vi "Receiving Modulated Audio.vi"() -> ()   [LabVIEW 2019]
doc: "This application receives an audio modulated signal from the other target by communicating with a TCP protocol. The signal is then outputed through the EMONA Communications Board for its demodulation. After being demodulated, the signal is reproduced on the headphones and inputed once again to the application. Finally the application displays the message received through the Message Chart."
uses:
  <vilib>/myRIO/Instrument Drivers/Onboard IO/AO Continuous/typedefs/AO Continuous Reference.ctl
  <vilib>/myRIO/Common/Instrument Driver Framework/Utilities/typedefs/myRIO Generic Hardware Reference.ctl
  <vilib>/myRIO/Common/Instrument Driver Framework/Utilities/typedefs/Hardware Version Enum.ctl
  <vilib>/myRIO/Common/Instrument Driver Framework/Utilities/typedefs/myRIO v1.0 Reference.ctl
  <vilib>/myRIO/Common/Instrument Driver Framework/Utilities/typedefs/Generic FPGA Reference.ctl
  <vilib>/myRIO/Common/Instrument Driver Framework/ELVIS III v1.0/AO Continuous/typedefs/AO Continuous Channels List.ctl
  <vilib>/myRIO/Common/Instrument Driver Framework/ELVIS III v1.0/AO Continuous/typedefs/ELVIS III v1.0 AO Continuous Channels Enum.ctl
  <vilib>/myRIO/Common/Instrument Driver Framework/ELVIS III v1.0/AO Continuous/typedefs/AO Continuous Channel Info.ctl
  <vilib>/userDefined/High Color/nirio_resource_hc.ctl
  <vilib>/myRIO/Instrument Drivers/Onboard IO/AI Block/typedefs/AI Block Reference.ctl
  <vilib>/myRIO/Common/Instrument Driver Framework/myRIO v1.0/AI Block/typedefs/AI Block Channels List.ctl
  <vilib>/myRIO/Common/Instrument Driver Framework/myRIO v1.0/AI Block/typedefs/AI Block Channels Enum.ctl
  <vilib>/myRIO/Common/Instrument Driver Framework/Utilities/typedefs/Analog Scaling Constants.ctl
  <vilib>/myRIO/Common/Instrument Driver Framework/ELVIS III v1.0/AO Continuous/vis/ELVIS III v1.1 Open AO (Continuous).vi
  <vilib>/myRIO/Common/Instrument Driver Framework/ELVIS III v1.0/AI Block/vis/ELVIS III v1.1 Open AI (N Samples).vi
  <vilib>/myRIO/Common/Instrument Driver Framework/Utilities/vis/Validate Channels.vi
  <vilib>/myRIO/Common/Instrument Driver Framework/ELVIS III v1.0/AO Continuous/vis/ELVIS III v1.0 Reserve AO Continuous.vi
  <vilib>/myRIO/Common/Instrument Driver Framework/ELVIS III v1.0/Resource Manager/vis/ELVIS III v1.0 Check For Different Banks.vi
  <vilib>/myRIO/Common/Instrument Driver Framework/ELVIS III v1.0/AI Block/vis/ELVIS III v1.0 AI Block Read.vi
  <vilib>/myRIO/Common/Instrument Driver Framework/ELVIS III v1.0/AI Block/vis/ELVIS III v1.0 Close AI Block.vi
  <vilib>/myRIO/Common/Instrument Driver Framework/ELVIS III v1.0/AO Continuous/vis/ELVIS III v1.1 Close AO Continuous.vi
  <vilib>/myRIO/Common/Instrument Driver Framework/myRIO v1.0/UART/vis/myRIO v1.0 Close UART.vi
  <vilib>/myRIO/Common/Instrument Driver Framework/ELVIS III v1.0/AO Continuous/vis/ELVIS III v1.0 Build MUX Configuration AO Continuous.vi
  <vilib>/myRIO/Common/Instrument Driver Framework/Utilities/vis/Sample Rate To Ticks.vi
  <vilib>/myRIO/Common/Instrument Driver Framework/ELVIS III v1.0/AI Block/vis/ELVIS III v1.0 Unreserve AI Block.vi
  <vilib>/myRIO/Common/Instrument Driver Framework/ELVIS III v1.0/AO Continuous/vis/ELVIS III v1.0 Unreserve AO Continuous.vi
  <vilib>/myRIO/Common/Instrument Driver Framework/ELVIS III v1.0/AI Block/vis/ELVIS III v1.0 Build MUX Configuration AI Block.vi
  <vilib>/Utility/VariantDataType/GetNumericInfo.vi
  <vilib>/Utility/error.llb/Error Cluster From Error Code.vi
  <vilib>/myRIO/Common/Instrument Driver Framework/ELVIS III v1.0/ELVIS III v1.1 Open.vi
  <vilib>/myRIO/Common/Instrument Driver Framework/ELVIS III v1.0/Resource Manager/vis/ELVIS III v1.0 Coerce AI Scaling.vi
  <vilib>/myRIO/Common/Instrument Driver Framework/ELVIS III v1.0/AI Block/vis/ELVIS III v1.0 Reserve AI Block.vi
  <vilib>/myRIO/Common/Instrument Driver Framework/ELVIS III v1.0/Resource Manager/vis/ELVIS III v1.0 Configure DMAs.vi
  <vilib>/myRIO/Common/Instrument Driver Framework/myRIO v1.0/myRIO v1.0 Close.vi
  <vilib>/myRIO/Common/Instrument Driver Framework/ELVIS III v1.0/Resource Manager/vis/ELVIS III v1.0 Reserve Channel List.vi
  <vilib>/myRIO/Common/Instrument Driver Framework/ELVIS III v1.0/AO Continuous/vis/ELVIS III v1.1 Stop AO Continuous.vi
  <vilib>/myRIO/Common/Instrument Driver Framework/myRIO v1.0/Resource Manager/vis/myRIO v1.0 Block Write Configuration.vi
  <vilib>/myRIO/Common/Instrument Driver Framework/ELVIS III v1.0/AI Block/vis/ELVIS III v1.0 AI Block Read Bank A.vi
  <vilib>/myRIO/Common/Instrument Driver Framework/ELVIS III v1.0/AI Block/vis/ELVIS III v1.0 AI Block Read Bank B.vi
  <vilib>/myRIO/Common/Instrument Driver Framework/ELVIS III v1.0/AO Continuous/vis/ELVIS III v1.0 AO Continuous Write.vi
  <vilib>/myRIO/Common/Instrument Driver Framework/ELVIS III v1.0/AO Continuous/vis/ELVIS III v1.1 Start AO Continuous.vi
  <vilib>/myRIO/Common/Instrument Driver Framework/ELVIS III v1.0/Resource Manager/vis/ELVIS III v1.0 Unreserve Channel List.vi
  <vilib>/myRIO/Common/Instrument Driver Framework/Utilities/vis/FPGA Ref Manager.vi
  <vilib>/myRIO/Common/Instrument Driver Framework/ELVIS III v1.0/ELVIS III v1.0 Reset FPGA.vi
  <vilib>/myRIO/Common/Instrument Driver Framework/myRIO v1.0/IRQ/vis/myRIO v1.0 IRQ Info FGV.vi
  <vilib>/myRIO/Common/Instrument Driver Framework/myRIO v1.0/IRQ/vis/myRIO v1.0 Timer IRQ Info FGV.vi
  <vilib>/myRIO/Common/Instrument Driver Framework/myRIO v1.0/IRQ/vis/myRIO v1.0 ISR Agent.vi
  <vilib>/myRIO/Instrument Drivers/Utilities/vis/Reset Index.vi
  <vilib>/myRIO/Common/Instrument Driver Framework/myRIO v1.0/Resource Manager/vis/myRIO v1.0 Block Write Resource Manager.vi
  <vilib>/myRIO/Instrument Drivers/Onboard IO/AI Block/vis/myRIO AI N Samples Open.xnode
  <vilib>/myRIO/Instrument Drivers/Onboard IO/AO Continuous/vis/myRIO AO Continuous Open.xnode
  <vilib>/myRIO/Instrument Drivers/Utilities/Utilities.lvlib
  <vilib>/myRIO/Instrument Drivers/Onboard IO/AI Block/AI Block.lvlib
  <vilib>/myRIO/Instrument Drivers/Onboard IO/AO Continuous/AO Continuous.lvlib
panel:
  out "Demodulator":string caption="Demodulator IP Address"
  out "Message":dbl[](graph)
  out "Signal":dbl[](graph) caption="Modulated Signal"
  out "Error Out":errorcluster
  in  "Stop":bool
  # "Receiving and Demodulating Audio"
  # "Explanation:\nThis application receives an audio modulated signal from the other target by communicating with a TCP protocol. The signal is then outputed through the EMONA Communications Board for its demodulation. After being demodulated, the signal is reproduced on the headphones and inputed once again to the application. Finally the application displays the message received through the Message Chart.\n \nThe audio from the target might sound lightly distortioned because of the modulation and demodulation process that was applied to the signal.\n \nInstructions:\n •  Make sure that you have uploaded at least one audio file to the Modulating target for its reproduction (use the Uploading Audio Files VI to do this).\n • Deploy the matching VIs (Sending and Receiving) to each target.\n • Enter the text from the indicator below into the Demodulator IP Address control from the Sending Modulated Audio.vi.\n • Run this VI again and afterwards run the other VI.\n • Try changing between songs and hearing the audio from both targets.\n • If you are not going to use any of the VIs from this project anymore, run the Remove Audio Files VI on the other target."
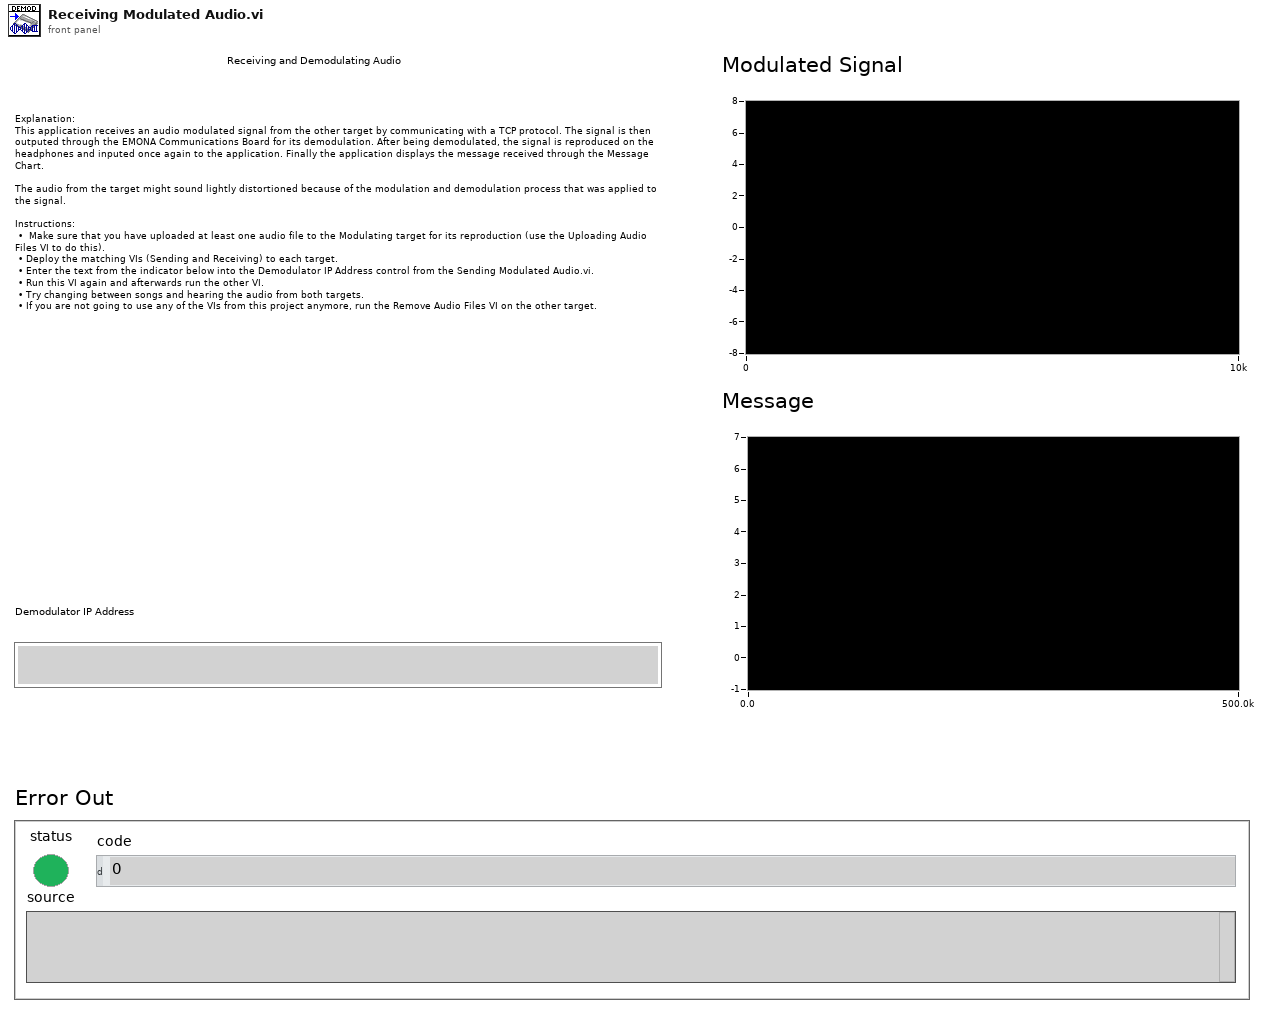
[diagram p1: front panel]
types:
  T1 = typedef "AO Continuous.lvlib/AO Continuous Reference.ctl" = cluster{"myRIO Reference":T2, "AO (Continuous) Channels List":T6, "Channel Info":T8}
  T2 = typedef "myRIO Generic Hardware Reference.ctl" = cluster{"myRIO Model":T3, "myRIO Hardware Reference":T4}
  T3 = typedef "Hardware Version Enum.ctl" = enum16{"Unknown", "myRIO-1900", "myRIO-1950", "roboRIO", "NI ELVIS RIO CM", "ELVIS III"}
  T4 = typedef "myRIO v1.0 Reference.ctl" = cluster{"Generic FPGA Reference":T5, "Allow multiple opens":bool}
  T5 = typedef "Generic FPGA Reference.ctl" = refnum<k20>
  T6 = typedef "AO Continuous Channels List.ctl" = T7[]
  T7 = typedef "ELVIS III v1.0 AO Continuous Channels Enum.ctl" = enum16{"Not Connected", "A/AO0 (Continuous)", "A/AO1 (Continuous)", "B/AO0 (Continuous)", "B/AO1 (Continuous)"}
  T8 = typedef "AO Continuous Channel Info.ctl" = cluster{"Channel Bitmask":u8[], "Channel Index":i32[], "Channel Number":u8}
  T9 = typedef "AI Block.lvlib/AI Block Reference.ctl" = cluster{"myRIO Reference":T2, "AI (N Samples) Channels List":T10, "AI (N Samples) Scaling Constants List":T12[]}
  T10 = typedef "AI Block Channels List.ctl" = T11[]
  T11 = typedef "AI Block Channels Enum.ctl" = enum16{"Not Connected", "A/AI0 (N Samples)", "A/AI1 (N Samples)", "A/AI2 (N Samples)", "A/AI3 (N Samples)", "A/AI4 (N Samples)", "A/AI5 (N Samples)", "A/AI6 (N Samples)", "A/AI7 (N Samples)", "A/AI0 (DIFF N Samples)", "A/AI1 (DIFF N Samples)", "A/AI2 (DIFF N Samples)", "A/AI3 (DIFF N Samples)", "B/AI0 (N Samples)", "B/AI1 (N Samples)", "B/AI2 (N Samples)", "B/AI3 (N Samples)", "B/AI4 (N Samples)", "B/AI5 (N Samples)", "B/AI6 (N Samples)", "B/AI7 (N Samples)", "B/AI0 (DIFF N Samples)", "B/AI1 (DIFF N Samples)", "B/AI2 (DIFF N Samples)", "B/AI3 (DIFF N Samples)"}
  T12 = typedef "Analog Scaling Constants.ctl" = cluster{"LSB Weight (Volts)":dbl, "Offset (Volts)":dbl, "Signed?":bool}
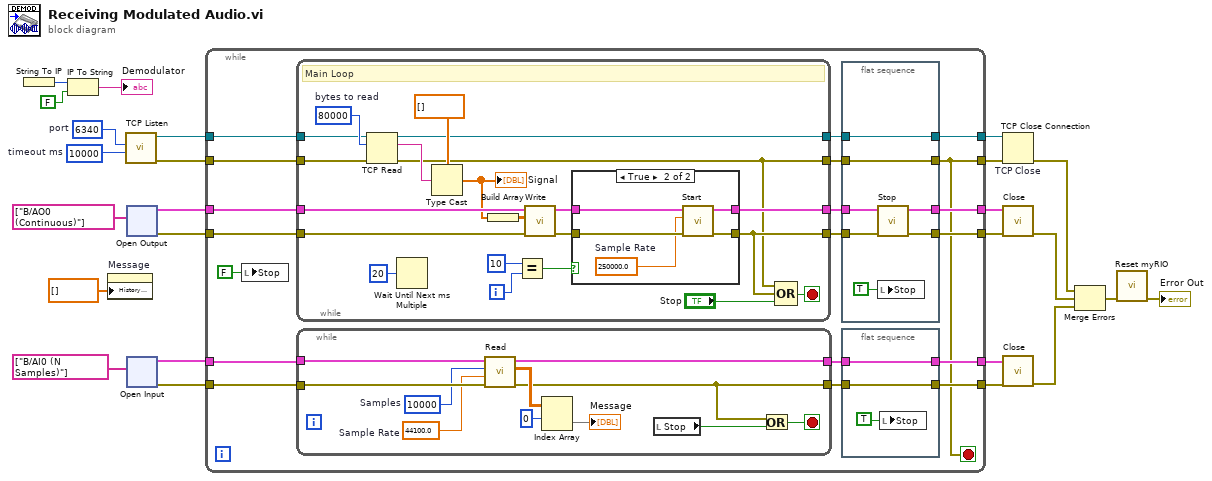
[diagram p0: block diagram]
diagram:
  w7 = 10000  # timeout ms
  w8 = u16 6340  # port
  n1 = String To IP() -> (0:w10:u32)  [unwired: 1 in]
  n2 = IP To String(1:FALSE ("dot notation? (F)"), 2:w10) -> (0:→"Demodulator":string)
  n3 = property on="Message" class="WFChart (strict)"("History Data"=dbl[] []) -> ()  [unwired: 2 in, 2 out]
  n4 = call <vilib>:"TCP Listen.vi"("timeout ms (wait forever: -1)"=w7, "port"=w8) -> ("error out"=w16:errorcluster, "connection ID"=w17:refnum<k5>)  [unwired: 5 in, 3 out]
  n5 = xnode "Open Output"("Channel Names"=tag[] ["B/AO0 (Continuous)"]) -> ("error out"=w20:errorcluster, "AO (Continuous) Ref Out"=w21:T1)  [unwired: 1 in]
  n6 = xnode "Open Input"("Channel Names"=tag[] ["B/AI0 (N Samples)"]) -> ("error out"=w25:errorcluster, "AI (N Samples) Ref Out"=w24:T9)  [unwired: 4 in]
  n7 = while {
    tunnel: w17 -> [w36]
    tunnel: [w34] -> w15
    tunnel: w16 -> [w35]
    tunnel: [w26] -> w14
    tunnel: w21 -> [w40]
    tunnel: [w37] -> w18
    tunnel: w20 -> [w39]
    tunnel: [w38] -> w19
    tunnel: w24 -> [w43]
    tunnel: [w41] -> w22
    tunnel: w25 -> [w44]
    tunnel: [w42] -> w23
    stop <- w26 stop-if-true
    n8 = local write "Stop"(FALSE ("Stop")) -> ()
    n9 = while {
      tunnel: w39 -> [w82]
      tunnel: [w75] -> w31
      tunnel: w40 -> [w83]
      tunnel: [w81] -> w32
      tunnel: w36 -> [w69]
      tunnel: w35 -> [w68]
      tunnel: [w71] -> w28
      tunnel: [w66] -> w27
      i -> [w77]
      stop <- w86 stop-if-true
      w70 = 80000  # bytes to read
      # "Main Loop"
      n10 = TCP Read(connection ID=w69, bytes to read=w70, error in (no error)=w68) -> (connection ID out=w71:refnum<k5>, data out=w73:string, error out=w66:errorcluster)  [unwired: 2 in]
      n11 = Wait Until Next ms Multiple(millisecond multiple=u32 20) -> ()  [unwired: 1 out]
      n12 = Type Cast(type=dbl[] [] ("chart"), x=w73) -> (*(type *) &x=w72:dbl[])
      "Signal" <- w72
      n13 = Build Array(w72) -> (w80:dbl[][])
      n14 = Equal?(x=10, y=w77) -> (x = y?=w78:bool)
      n15 = call <vilib>:"Write.vi"("error in (no error)"=w82, "Data To Write"=w80, "AO (Continuous) Ref In"=w83) -> ("error out"=w84:errorcluster, "AO (Continuous) Ref Out"=w85:T1)  [unwired: 7 in]
      n16 = case shown="True" w78 {
        tunnel: w85 -> [w88 w93]
        tunnel: w84 -> [w87 w92]
        tunnel: [w88 w91] -> w81
        tunnel: [w87 w90] -> w75
        frame False {
        }
        frame True {
          w89 = 250000.0  # Sample Rate
          n17 = call <vilib>:"Start.vi"("error in (no error)"=w92, "Sample Rate"=w89, "AO (Continuous) Ref In"=w93) -> ("error out"=w90:errorcluster, "AO (Continuous) Ref Out"=w91:T1)  [unwired: 7 in]
        }
      }
      n18 = Compound Arithmetic op=OR(w66, w75, "Stop") -> (w86:bool)
    }
    n19 = while {
      tunnel: w43 -> [w65]
      tunnel: [w61] -> w30
      tunnel: w44 -> [w64]
      tunnel: [w56] -> w29
      stop <- w63 stop-if-true
      w57 = u32 10000  # Samples
      w58 = 44100.0  # Sample Rate
      n20 = call <vilib>:"Read.vi"("error in (no error)"=w64, "Sample Rate [Hz]"=w58, "Number of Samples"=w57, "AI (N Samples) Ref In"=w65) -> ("error out"=w56:errorcluster, "Values"=w60:dbl[][], "AI (N Samples) Ref Out"=w61:T9)  [unwired: 5 in]
      n21 = Index Array(array=w60, index (row)=0) -> (element=→"Message":dbl[])  [unwired: 1 in]
      n22 = local read "Stop"() -> (w62:bool)
      n23 = Or(x=w56, y=w62) -> (x .or. y?=w63:bool)
    }
    n24 = flat-sequence {
      tunnel: w32 -> [w51]
      tunnel: w31 -> [w50]
      tunnel: [w53] -> w38
      tunnel: [w52] -> w37
      tunnel: w28 -> [w49]
      tunnel: [w49] -> w34
      tunnel: w27 -> [w48]
      tunnel: [w48] -> w26
      frame #0 {
        n25 = call <vilib>:"Stop.vi"("error in (no error)"=w50, "AO (Continuous) Ref In"=w51) -> ("error out"=w53:errorcluster, "AO (Continuous) Ref Out"=w52:T1)  [unwired: 8 in]
        n26 = local write "Stop"(TRUE ("Stop")) -> ()
      }
    }
    n27 = flat-sequence {
      tunnel: w30 -> [w47]
      tunnel: [w47] -> w41
      tunnel: w29 -> [w46]
      tunnel: [w46] -> w42
      frame #0 {
        n28 = local write "Stop"(TRUE ("Stop")) -> ()
      }
    }
  }
  n29 = TCP Close Connection "TCP Close"(connection ID=w15, error in (no error)=w14) -> (error out=w1:errorcluster)  [unwired: 1 in, 1 out]
  n30 = call <vilib>:"Close.vi"("error in (no error)"=w19, "AO (Continuous) Ref In"=w18) -> ("error out"=w3:errorcluster)  [unwired: 9 in]
  n31 = call <vilib>:"Close.vi"("error in (no error)"=w23, "AI (N Samples) Ref In"=w22) -> ("error out"=w2:errorcluster)  [unwired: 9 in]
  n32 = Merge Errors(w1, w3, w2) -> (w4:errorcluster)
  n33 = call <vilib>:"Reset myRIO.vi"("error in (no error)"=w4) -> ("error out"=→"Error Out":errorcluster)  [unwired: 10 in]
